vi "Error Engine - Find Data Folder.vi"(0 "Target Folder":string="Data", 3 "Error In":errorcluster) -> (7 "Target Folder Path":path, 9 "Pass?":bool, 10 "Error Out":errorcluster)   [LabVIEW 2023, in "Error_Engine_Actor.lvlib" / "Error_Emgime_Class.lvclass"]
uses:
  Error_Emgime_Class.lvclass
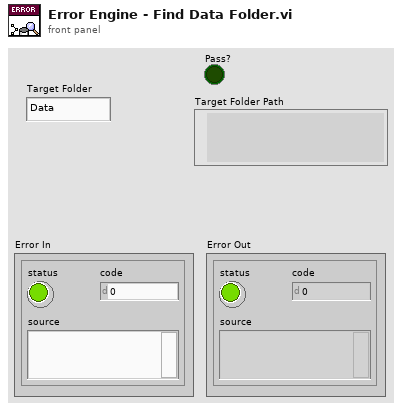
[diagram p1: front panel]
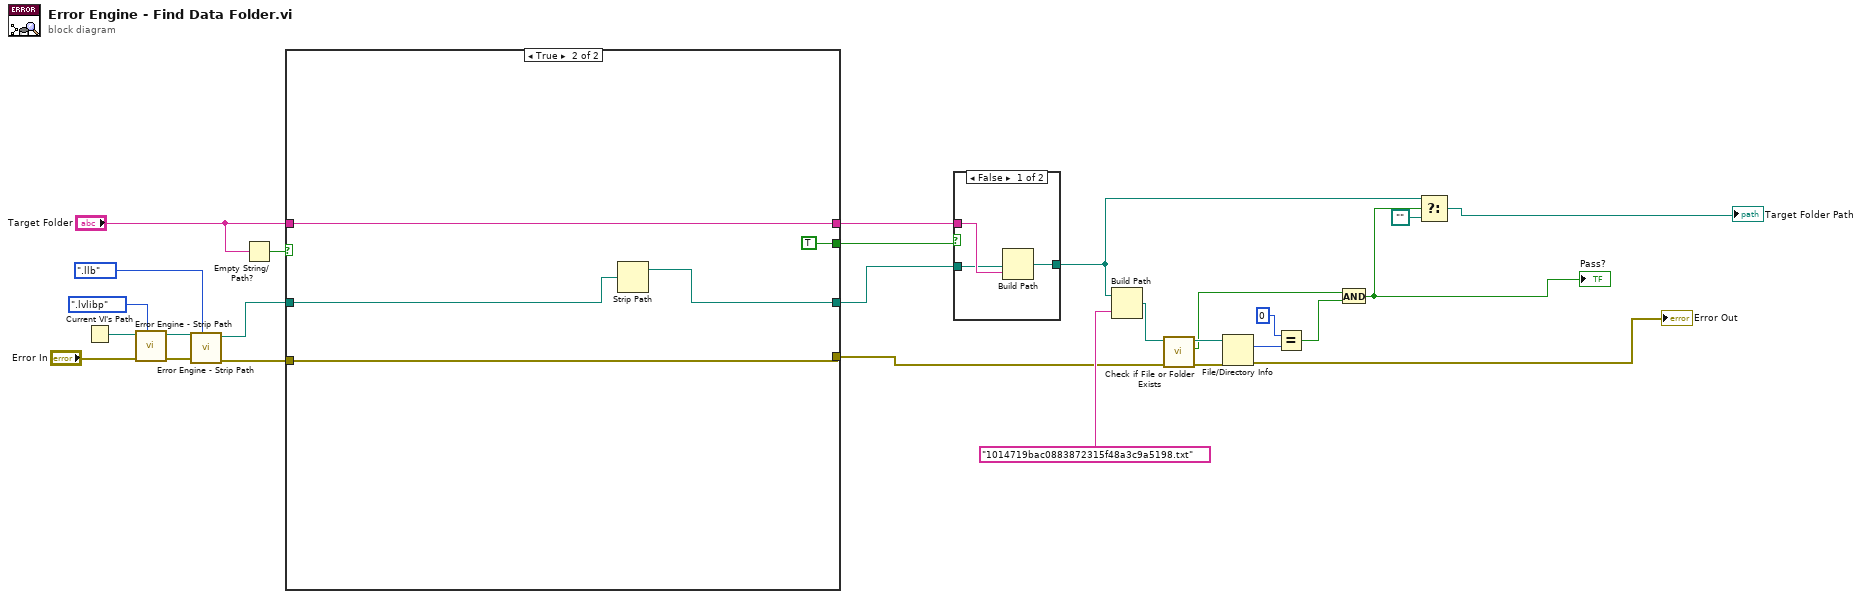
[diagram p0: block diagram]
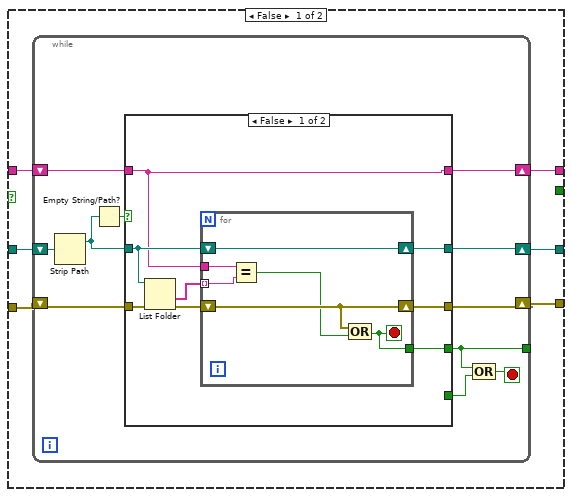
[diagram p3: hidden frame]
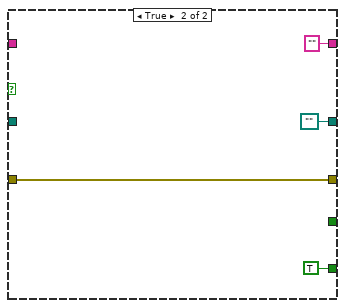
[diagram p4: hidden frame]
diagram:
  n1 = Current VI's Path() -> (path=w26:path)
  n2 = call "Error Engine - Strip Path.vi"("Strip Lib App Types"=enum16{".lvlibp", ".exe", ".llb"}.".lvlibp", "error in (no error)"="Error In", "File Path In"=w26) -> ("error out"=w24:errorcluster, "Stripped File Path"=w23:path)  [unwired: 7 in]
  n3 = call "Error Engine - Strip Path.vi"("Strip Lib App Types"=enum16{".lvlibp", ".exe", ".llb"}.".llb", "error in (no error)"=w24, "File Path In"=w23) -> ("error out"=w22:errorcluster, "Stripped File Path"=w20:path)  [unwired: 7 in]
  n4 = Empty String/Path?(string/path="Target Folder") -> (empty?=w3:bool)
  n5 = case shown="True" w3 {
    tunnel: w22 -> [w33 w67]
    tunnel: w20 -> [w32 w65]
    tunnel: "Target Folder" -> [w31 w66]
    tunnel: [w30 w67] -> w9
    tunnel: [w29 w66] -> w8
    tunnel: [w28 w64] -> w7
    tunnel: [_ TRUE] -> w1
    frame False {
      n6 = while {
        shift-right: [w41] -> w28
        shift-left: w32 -> [w44]
        shift-right: [w40] -> w30
        shift-left: w33 -> [w43]
        shift-right: [w37] -> w29
        shift-left: w31 -> [w42]
        tunnel: [w36] -> _
        stop <- w34 stop-if-true
        n7 = Strip Path(path=w44) -> (stripped path=w39:path)  [unwired: 1 out]
        n8 = Empty String/Path?(string/path=w39) -> (empty?=w38:bool)
        n9 = case shown="False" w38 {
          tunnel: w43 -> [w52 w62]
          tunnel: w42 -> [w45 _]
          tunnel: [w49 path "" ("stripped path")] -> w41
          tunnel: [w48 w62] -> w40
          tunnel: [w47 _] -> w36
          tunnel: w39 -> [w46 _]
          tunnel: [_ TRUE] -> w35
          tunnel: [w45 "" ("Target Folder")] -> w37
          frame False {
            n10 = List Folder(path=w46, error in=w52) -> (folder names=w50:string[], error out=w51:errorcluster)  [unwired: 2 in, 2 out]
            n11 = for {
              shift-right: [w56] -> w48
              shift-left: w51 -> [w56]
              tunnel: w50 -> [w58] mode=indexing
              tunnel: w45 -> [w57]
              shift-right: [w54] -> w49
              shift-left: w46 -> [w54]
              tunnel: [w53] -> w47
              stop <- w53 stop-if-true
              n12 = Equal?(x=w57, y=w58) -> (x = y?=w55:bool)
              n13 = Compound Arithmetic op=OR(w56, w55) -> (w53:bool)
            }
          }
          frame True {
          }
        }
        n14 = Compound Arithmetic op=OR(w36, w35) -> (w34:bool)
      }
    }
    frame True {
      n15 = Strip Path(path=w65) -> (stripped path=w64:path)  [unwired: 1 out]
    }
  }
  n16 = case shown="False" w1 {
    tunnel: [w70 w71] -> w11
    tunnel: w8 -> [w69 _]
    tunnel: w7 -> [w68 w71]
    frame False {
      n17 = Build Path(base path=w68, name or relative path=w69) -> (appended path=w70:path)
    }
    frame True {
    }
  }
  n18 = Build Path(base path=w11, name or relative path="1014719bac0883872315f48a3c9a5198.txt") -> (appended path=w18:path)
  n19 = call <vilib>:"Check if File or Folder Exists.vi"("error in (no error)"=w9, "path"=w18) -> ("error out"=w17:errorcluster, "file or folder exists?"=w12:bool, "dup path"=w16:path)  [unwired: 7 in]
  n20 = File/Directory Info(path=w16, error in=w17) -> (size=w15:i64, error out=→"Error Out":errorcluster)  [unwired: 5 out]
  n21 = Equal?(x=i64 0, y=w15) -> (x = y?=w13:bool)
  n22 = And(x=w12, y=w13) -> (x .and. y?=w5:bool)
  "Pass?" <- w5
  n23 = Select(t=w11, s=w5, f=path "") -> (s? t:f=→"Target Folder Path":path)
